vi "loopindexing.vi"() -> ()   [LabVIEW 2015]
panel:
  out "Number of iterations":i32
  in  "stop":bool
  out "Array 2":i16[](array[numeric])
  in  "Array":i16[](array[numeric])
  # "Array original"
  # "Valores para los cuales es menor o igual a 10"
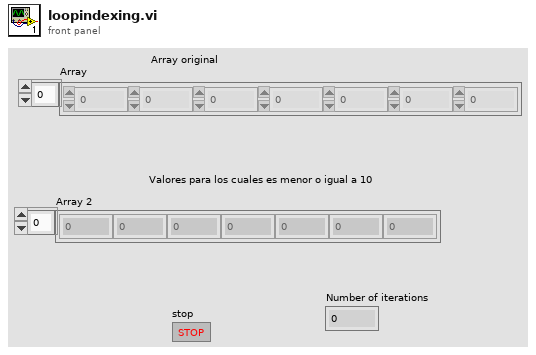
[diagram p1: front panel]
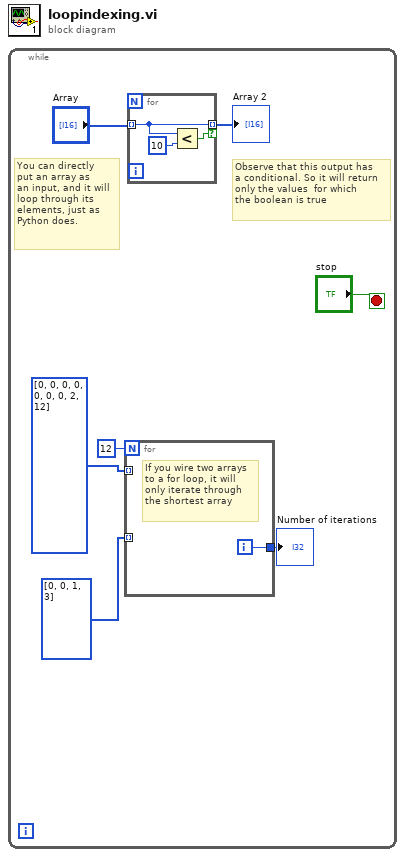
[diagram p0: block diagram]
diagram:
  n1 = while {
    stop <- "stop" stop-if-true
    # "Observe that this output has\na conditional. So it will return\nonly the values  for which\nthe boolean is true"
    # "You can directly\nput an array as\nan input, and it will\nloop through its\nelements, just as\nPython does."
    n2 = for {
      N: 12 -> [_]
      tunnel: [w8] -> w4
      tunnel: i32[] [0, 0, 0, 0, 0, 0, 0, 2, 12] -> [_] mode=indexing
      tunnel: i32[] [0, 0, 1, 3] -> [_] mode=indexing
      i -> [w8]
      # "If you wire two arrays\nto a for loop, it will \nonly iterate through\nthe shortest array"
    }
    "Number of iterations" <- w4
    n3 = for {
      tunnel: "Array" -> [w10] mode=indexing
      tunnel: [w10] -> w6 mode=indexing if=w9
      n4 = Less?(x=w10, y=i16 10) -> (x < y?=w9:bool)
    }
    "Array 2" <- w6
  }
